vi "Sequence Get Triggers.vi"(11 "Excel file in":refnum<class "NI_report.lvclass">) -> (0 "Valid?":bool=TRUE, 2 "Triggers":T1[](array[typedef]))   [LabVIEW 2015]
uses:
  <vilib>/Utility/NIReport.llb/NI_report.lvclass
  Test Sequence Trigger.ctl
  Sensors/Sensor Enum.ctl
  <vilib>/addons/_office/excel.llb/Excel Get Data ([str]).vi
  <vilib>/addons/_office/NI_ReportGenerationToolkit.lvlib
  <vilib>/Utility/NIReport.llb/Excel/NI_Excel.lvclass
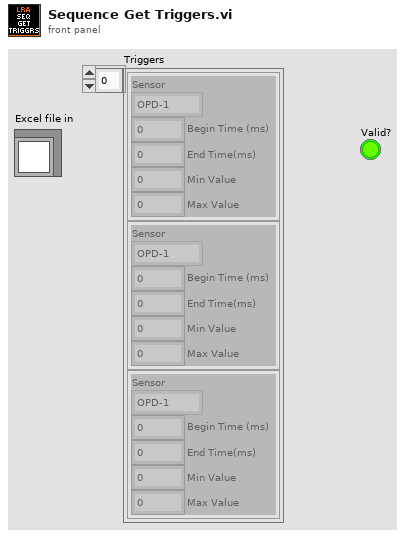
[diagram p1: front panel]
types:
  T1 = typedef "Test Sequence Trigger.ctl" = cluster{"Sensor":T2, "Begin Time (ms)":dbl, "End Time(ms)":dbl, "Min Value":dbl, "Max Value":dbl}
  T2 = typedef "Sensor Enum.ctl" = enum16{"OPD-1", "OPD-2", "OPD-3", "OTC-1", ""}
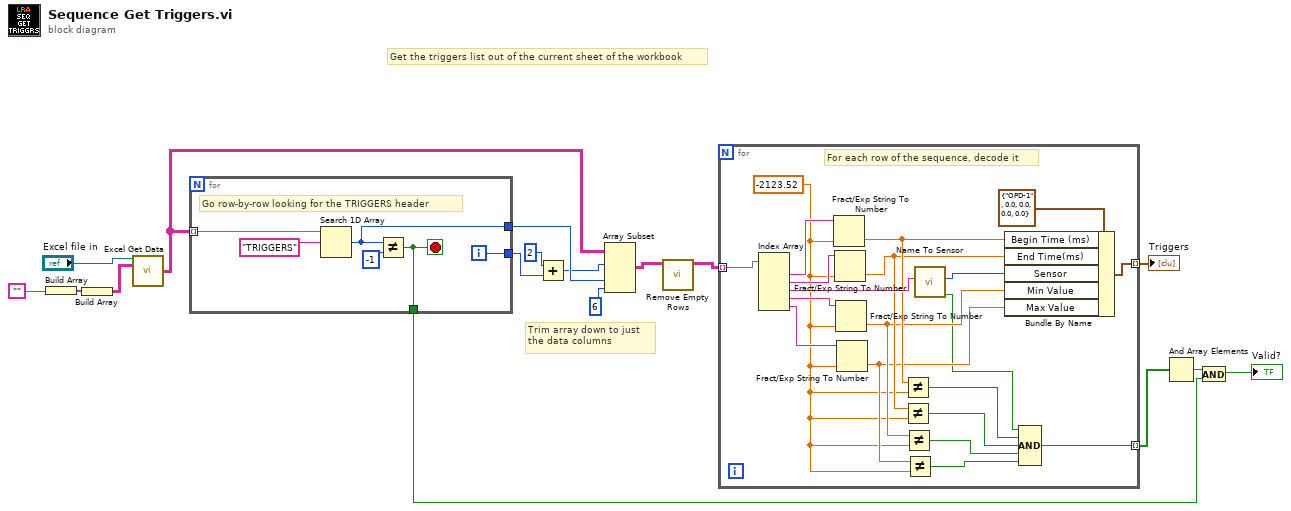
[diagram p0: block diagram]
diagram:
  # "Trim array down to just \nthe data columns"
  # "Get the triggers list out of the current sheet of the workbook"
  n1 = Build Array("") -> (w15:string[])
  n2 = Build Array(w15) -> (w14:string[][])
  n3 = call-poly <vilib>:"Excel Get Data.vi"("report in"="Excel file in", "data type"=w14) -> ("data"=w13:string[][])  [unwired: 11 in, 2 out]
  n4 = for {
    tunnel: w13 -> [w23] mode=indexing
    tunnel: [w20] -> w11
    tunnel: [w19] -> w9
    tunnel: [w18] -> w5
    i -> [w19]
    stop <- w18 stop-if-true
    # "Go row-by-row looking for the TRIGGERS header"
    n5 = Search 1D Array(1D array=w23, element="TRIGGERS") -> (index of element=w20:i32)  [unwired: 1 in]
    n6 = Not Equal?(x=w20, y=-1) -> (x != y?=w18:bool)
  }
  n7 = Add(x=2, y=w9) -> (x+y=w8:i32)
  n8 = Array Subset(array=w13, index (row)=w8, index (col)=w11, length (col)=6 ("length")) -> (w2:string[][])  [unwired: 1 in]
  n9 = call "Remove Empty Rows.vi"("Array in"=w2) -> ("Array out"=w1:string[][])  [unwired: 10 in]
  n10 = for {
    tunnel: w1 -> [w43] mode=indexing
    tunnel: [w25] -> w4 mode=indexing
    tunnel: [w24] -> w3 mode=indexing
    w31 = -2123.52
    # "For each row of the sequence, decode it"
    n11 = Index Array(array=w43) -> (element #1=w41:string, element #2=w40:string, element #3=w39:string, element #4=w37:string, element #5=w36:string)  [unwired: 5 in]
    n12 = Fract/Exp String To Number(string=w41, default (0 dbl)=w31) -> (number=w35:dbl)  [unwired: 2 in, 1 out]
    n13 = Fract/Exp String To Number(string=w40, default (0 dbl)=w31) -> (number=w34:dbl)  [unwired: 2 in, 1 out]
    n14 = Fract/Exp String To Number(string=w37, default (0 dbl)=w31) -> (number=w33:dbl)  [unwired: 2 in, 1 out]
    n15 = Fract/Exp String To Number(string=w36, default (0 dbl)=w31) -> (number=w32:dbl)  [unwired: 2 in, 1 out]
    n16 = Not Equal?(x=w35, y=w31) -> (x != y?=w29:bool)
    n17 = Not Equal?(x=w34, y=w31) -> (x != y?=w28:bool)
    n18 = Not Equal?(x=w33, y=w31) -> (x != y?=w27:bool)
    n19 = Not Equal?(x=w32, y=w31) -> (x != y?=w26:bool)
    n20 = call "Name To Sensor.vi"("Sensor Name"=w39) -> ("Found?"=w30:bool, "Sensor Enum"=w38:T2)  [unwired: 9 in]
    n21 = Bundle By Name(cluster=T1 {"Sensor"=enum."OPD-1", "Begin Time (ms)"=0.0, "End Time(ms)"=0.0, "Min Value"=0.0, "Max Value"=0.0} ("Cluster"), "Begin Time (ms)"=w35, "End Time(ms)"=w34, "Sensor"=w38, "Min Value"=w33, "Max Value"=w32) -> (w24:T1)
    n22 = Compound Arithmetic op=AND(w30, w29, w28, w27, w26) -> (w25:bool)
  }
  "Triggers" <- w3
  n23 = And Array Elements(Boolean array=w4) -> (logical AND=w7:bool)
  n24 = And(x=w7, y=w5) -> (x .and. y?=→"Valid?":bool)
